vi "Housekeeping.vi"(8 "error in (no error)":errorcluster, 11 "CIFPlugin in":refnum<class "Template_Plugin.lvclass">) -> (0 "error out":errorcluster, 3 "CIFPlugin out":refnum<class "Template_Plugin.lvclass">)   [LabVIEW 2021, in "Template_Plugin.lvclass"]
uses:
  Template_Plugin.lvclass
  C:/Program Files/National Instruments/LabVIEW 2021/vi.lib/CIF Foundation/CIF Core/CIFCore/Class/CIFCorePlugin.lvclass
  <vilib>/CIF Foundation/CIF Core/CIFCore/Class/Typedef/Energized States.ctl
  <vilib>/CIF Foundation/CIF Core/CIFCore/Class/CIFCorePlugin.lvclass/CIFCorePlugin.ctl
  <vilib>/CIF Foundation/CIF Utilities/Statistics/I64/Stats_I64_CIF_U.lvclass/Stats_I64_CIF_U.ctl
  Template_Plugin.lvclass/Template_Plugin.ctl
  <vilib>/CIF Foundation/CIF Core/Channels/CIFChannelMng/CIFChannelMng.lvclass/CIFChannelMng.ctl
  <vilib>/CIF Foundation/CIF Channels Core/CIFChannels/CIFChannels.lvclass/CIFChannels.ctl
  <vilib>/CIF Foundation/CIF Core/CIFCore/Class/Accessors/Timestamps/Write Housekeeping TS.vi
  <vilib>/CIF Foundation/CIF Utilities/Time/System Time/Get System Time.vi
  <vilib>/CIF Foundation/CIF Utilities/Statistics/I64/X1 minus X0.vi
  <vilib>/CIF Foundation/CIF Utilities/Statistics/I64/Cyclic.vi
  <vilib>/CIF Foundation/CIF Core/CIFCore/Class/Benchmarking/Reset Delay.vi
  <vilib>/CIF Foundation/CIF Core/CIFCore/Class/Accessors/Timestamps/Read Execute TS.vi
  <vilib>/CIF Foundation/CIF Core/CIFCore/Class/Accessors/Timestamps/Read Housekeeping TS.vi
  <vilib>/CIF Foundation/CIF Core/CIFCore/Class/Accessors/Timestamps/Read Sleep TS.vi
  <vilib>/CIF Foundation/CIF Core/CIFCore/Class/Accessors/Timestamps/Read Target Wake TS.vi
  <vilib>/CIF Foundation/CIF Core/CIFCore/Class/SubVIs/Refresh Stats.vi
  <vilib>/CIF Foundation/CIF Core/CIFCore/Class/SubVIs/OOB/Receive/Read Clock Map.vi
  <vilib>/CIF Foundation/CIF Core/CIFCore/Class/SubVIs/OOB/Receive/Read Connections.vi
  <vilib>/CIF Foundation/CIF Core/Channels/CIFChannelMng/Core/Send Channel List Update.vi
  <vilib>/CIF Foundation/CIF Core/Channels/CIFChannelMng/SubVIs/Connect Channel.vi
  <vilib>/CIF Foundation/CIF Core/CIFCore/Class/SubVIs/OOB/Receive/Read Forces.vi
  <vilib>/CIF Foundation/CIF Core/Channels/CIFChannelMng/SubVIs/Force Channel.vi
  <vilib>/CIF Foundation/CIF Core/Channels/CIFChannelMng/SubVIs/Add FIFO Publisher.vi
  <vilib>/CIF Foundation/CIF Core/CIFCore/Class/SubVIs/OOB/Receive/Read Publisher Instance.vi
  <vilib>/CIF Foundation/CIF Core/Channels/CIFChannelMng/Core/Send Publisher Instance Return.vi
  <vilib>/CIF Foundation/CIF Core/Channels/CIFChannelMng/SubVIs/Remove FIFO Publisher.vi
  <vilib>/CIF Foundation/CIF Core/CIFCore/Class/SubVIs/OOB/Read Core OOB RX.vi/a31a91a9-4107-4750-8e0d-44486e9a3a34.vi
  <vilib>/CIF Foundation/CIF Core/CIFCore/Class/SubVIs/OOB/Update Status from Benchmarks.vi
  <vilib>/CIF Foundation/CIF Core/CIFCore/Class/SubVIs/OOB/Send Core OOB TX.vi/074d8088-3ad4-4fdc-9542-b009f1b06b72.vi
  OOB Comm/Read Comm to Main.vi/525c214c-2a6b-4e7b-b3ce-0ad96b412d2f.vi
  OOB Comm/Read Comm to Main.vi/4efb0375-f1de-4191-b03f-44d34e6646cb.vi
  OOB Comm/Send Cyclic to gRPC.vi/0c0f428d-7269-422d-ba27-f9d6fa7232ec.vi
  <vilib>/CIF Foundation/CIF Core/CIFCore/Class/Accessors/Read Refresh.vi
  <vilib>/CIF Foundation/CIF Utilities/Time/System Time/LabVIEW Time to TAI Time.vi
  <vilib>/CIF Foundation/CIF Utilities/Statistics/I64/X1 minus X0.vi/dfabcf33-0dbc-4041-80a5-3dc0c86d2989.vi
  <vilib>/CIF Foundation/CIF Utilities/Statistics/I64/Cyclic.vi/dfabcf33-0dbc-4041-80a5-3dc0c86d2989.vi
  <vilib>/CIF Foundation/CIF Core/Channels/CIFChannelMng/Core/Send Channel List Update.vi/463ebf4c-8748-40f9-8ad3-9e61c16a01a6.vi
  <vilib>/CIF Foundation/CIF Core/Channels/CIFChannelMng/Utilities/Get Channel Index by Name.vi
  <vilib>/CIF Foundation/CIF Channels Core/CIFChannels/Accessors/Read Channel State.vi
  <vilib>/CIF Foundation/CIF Channels Core/CIFChannels/Accessors/Read Tag Forced.vi
  <vilib>/CIF Foundation/CIF Core/Channels/CIFChannelMng/SubVIs/Add Error Channel Manager.vi
  <vilib>/CIF Foundation/CIF Core/Channels/CIFChannelMng/Core/Send Publisher Instance Return.vi/9db40550-ae0b-4108-a32d-02e81b824dbe.vi
  <vilib>/CIF Foundation/CIF Core/Channels/CIFChannelMng/SubVIs/Get Original FIFO Channel Name.vi
  <vilib>/CIF Foundation/CIF CIPC/SubVIs/Wait For N Elements Available.vi
  <vilib>/CIF Foundation/CIF CIPC/SubVIs/Check Error.vi
  <vilib>/CIF Foundation/CIF CIPC/SubVIs/Get dll Path.vi
  <vilib>/CIF Foundation/CIF CIPC/SubVIs/Get Element Read Position.vi
  <vilib>/CIF Foundation/CIF CIPC/SubVIs/Set Element Read Position.vi
  <vilib>/CIF Foundation/CIF Utilities/Statistics/I64/Get Stats.vi
  <vilib>/CIF Foundation/CIF CIPC/SubVIs/Notify Of New Write.vi
  <vilib>/CIF Foundation/CIF CIPC/SubVIs/Get Element Write Position.vi
  <vilib>/CIF Foundation/CIF Utilities/Statistics/I64/X1 minus X0.vi/dfabcf33-0dbc-4041-80a5-3dc0c86d2989.vi/9eb60a9a-770f-4d2d-8b3f-8465c267ecc9.vi
  <vilib>/CIF Foundation/CIF Utilities/Statistics/I64/Cyclic.vi/dfabcf33-0dbc-4041-80a5-3dc0c86d2989.vi/9eb60a9a-770f-4d2d-8b3f-8465c267ecc9.vi
  <vilib>/CIF Foundation/CIF Channels Core/ChannelCommon/Utilities/Add Error.vi
  <vilib>/CIF Foundation/CIF Utilities/Errors/Append Error Location.vi
  <vilib>/CIF Foundation/CIF CIPC/SubVIs/Get Element Info Variant.vi
  <vilib>/Utility/error.llb/Trim Whitespace.vi
  <vilib>/Utility/error.llb/Error Cluster From Error Code.vi
  <vilib>/CIF Foundation/CIF Channels Core/CIFChannels/Core/Set Force.vi
  <vilib>/CIF Foundation/CIF Core/CIFCore/Class/CIFCorePlugin.lvclass
  <vilib>/CIF Foundation/CIF Channels Core/CIFChannels/CIFChannels.lvclass
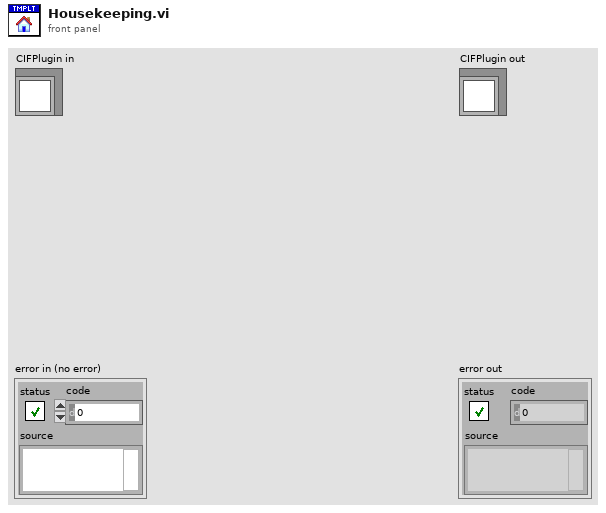
[diagram p1: front panel]
types:
  T1 = typedef "CIFCorePlugin.lvclass/Energized States.ctl" = enum16{"Listen", "Prepare", "Execute", "Housekeep", "Cleanup", "Destroy"}
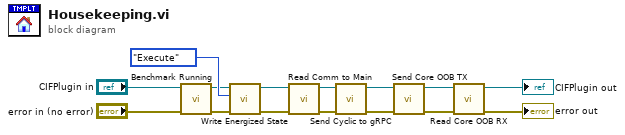
[diagram p0: block diagram]
diagram:
  n1 = call <vilib>:"Benchmark Running.vi"("error in (no error)"="error in (no error)", "CIFCorePlugin in"="CIFPlugin in") -> ("error out"=w11:errorcluster, "CIFCorePlugin out"=w6:refnum<class "Template_Plugin.lvclass">)  [unwired: 8 in]
  n2 = call <vilib>:"Write Energized State.vi"("error in (no error)"=w11, "Energized State"=Energized_States."Execute", "CIFCorePlugin in"=w6) -> ("error out"=w10:errorcluster, "CIFCorePlugin out"=w8:refnum<class "Template_Plugin.lvclass">)  [unwired: 7 in]
  n3 = call "Read Comm to Main.vi"("error in (no error)"=w10, "CIFTemplatePlugin in"=w8) -> ("error out"=w12:errorcluster, "CIFTemplatePlugin out"=w13:refnum<class "Template_Plugin.lvclass">)  [unwired: 8 in]
  n4 = call "Send Cyclic to gRPC.vi"("error in (no error)"=w12, "CIFTemplatePlugin in"=w13) -> ("error out"=w14:errorcluster, "CIFTemplatePlugin out"=w9:refnum<class "Template_Plugin.lvclass">)  [unwired: 8 in]
  n5 = call <vilib>:"Send Core OOB TX.vi"("error in (no error)"=w14, "CIFCorePlugin in"=w9) -> ("error out"=w15:errorcluster, "CIFCorePlugin out"=w5:refnum<class "Template_Plugin.lvclass">)  [unwired: 8 in]
  n6 = call <vilib>:"Read Core OOB RX.vi"("error in (no error)"=w15, "CIFCorePlugin in"=w5) -> ("error out"=→"error out":errorcluster, "CIFCorePlugin out"=→"CIFPlugin out":refnum<class "Template_Plugin.lvclass">)  [unwired: 8 in]
